vi "Decode Return Codes.vi"(10 "Return Codes":u8[](array[numeric]) format="%08b") -> (1 "Invalid Code?":bool, 2 "Subscription Success":T1[](array[typedef]))   [LabVIEW 2013, in "MQTT_Control_Packets.lvlib" / "SUBACK.lvclass"]
uses:
  SUBACK.lvclass
  Subscription Success Code.ctl
  ControlPacket/QualityOfService -- enum.ctl
  ControlPacket/ControlPacket.lvclass
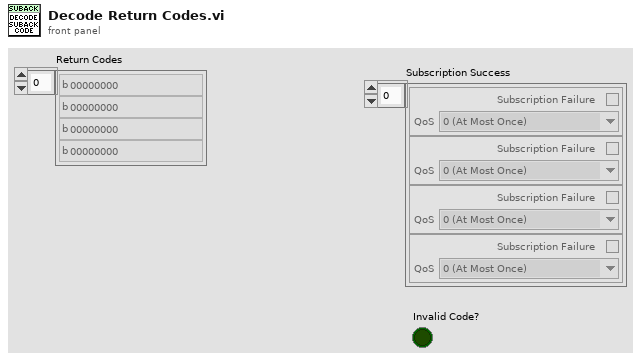
[diagram p1: front panel]
types:
  T1 = typedef "MQTT_Control_Packets.lvlib/SUBACK.lvclass/Subscription Success Code.ctl" = cluster{"Subscription Failure":bool, "QoS":T2}
  T2 = typedef "MQTT_Control_Packets.lvlib/ControlPacket.lvclass/QualityOfService -- enum.ctl" = enum16{"0 (At Most Once)", "1 (At Least Once)", "2 (Exactly Once)"}
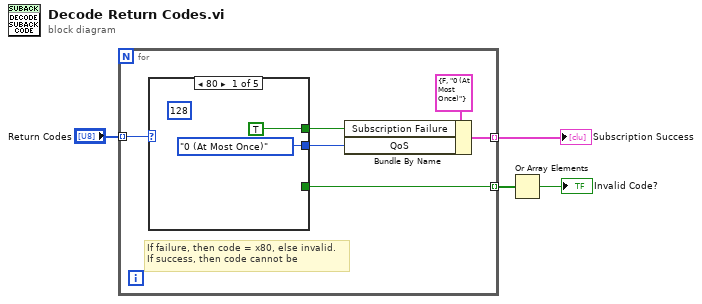
[diagram p0: block diagram]
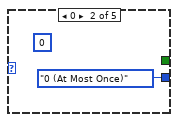
[diagram p2: hidden frame]
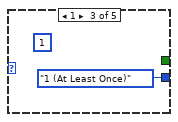
[diagram p3: hidden frame]
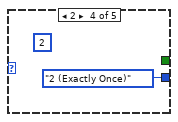
[diagram p4: hidden frame]
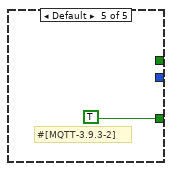
[diagram p5: hidden frame]
diagram:
  n1 = for {
    tunnel: "Return Codes" -> [w8] mode=indexing
    tunnel: [w9] -> w3 mode=indexing
    tunnel: [w5] -> w2 mode=indexing
    # "If failure, then code = x80, else invalid.\nIf success, then code cannot be"
    n2 = case shown="80" w8 {
      tunnel: [QualityOfService_--_enum."0 (At Most Once)" ("QoS") QualityOfService_--_enum."0 (At Most Once)" ("QoS") QualityOfService_--_enum."1 (At Least Once)" ("QoS") QualityOfService_--_enum."2 (Exactly Once)" ("QoS") _] -> w7
      tunnel: [TRUE _ _ _ _] -> w6
      tunnel: [_ _ _ _ TRUE] -> w5
      frame 128 {
        (unwired) u8 128 ("y")
      }
      frame 0 {
        (unwired) u8 0 ("y")
      }
      frame 1 {
        (unwired) u8 1 ("y")
      }
      frame 2 {
        (unwired) u8 2 ("y")
      }
      frame Default {
        # "#[MQTT-3.9.3-2]"
      }
    }
    n3 = Bundle By Name(cluster=T1 {"Subscription Failure"=FALSE, "QoS"=enum."0 (At Most Once)"} ("Topic Subscription"), "Subscription Failure"=w6, "QoS"=w7) -> (w9:T1)
  }
  "Subscription Success" <- w3
  n4 = Or Array Elements(Boolean array=w2) -> (logical OR=→"Invalid Code?":bool)
